vi "Event-Driven State Machine - Inject Error.vi"() -> ()   [LabVIEW 2020]
uses:
  support/States.ctl
  support/State Machine Data.ctl
  <vilib>/DAQmx/read.llb/DAQmx Read (Analog 2D DBL NChan NSamp).vi
  <vilib>/DAQmx/write.llb/DAQmx Write (Analog DBL 1Chan 1Samp).vi
  <vilib>/DAQmx/create/channels.llb/DAQmx Create Channel (AI-Voltage-Basic).vi
  <vilib>/DAQmx/configure/timing.llb/DAQmx Timing (Sample Clock).vi
  <vilib>/DAQmx/miscellaneous.llb/DAQmx Fill In Error Info.vi
  <vilib>/Utility/file.llb/Write Delimited Spreadsheet (DBL).vi
  <vilib>/DAQmx/create/channels.llb/DAQmx Create Channel (AO-Voltage-Basic).vi
panel:
  in  "AO Voltage Channel":tag="PCI-6221/ao1"
  in  "Generate Stimulus":bool
  out "Threshold exceeded?":bool
  in  "Acquire":bool
  in  "Samples per channel":i32=100
  in  "Sample Rate (Hz)":dbl=1000.0
  in  "AI Voltage Channel":tag="PCI-6221/ai0, PCI-6221/ai2:3"
  in  "Threshold (rms)":dbl=1.0
  in  "Clear":bool
  in  "Exit":bool
  out "Graph":dbl[][](graph)
  # "Analysis"
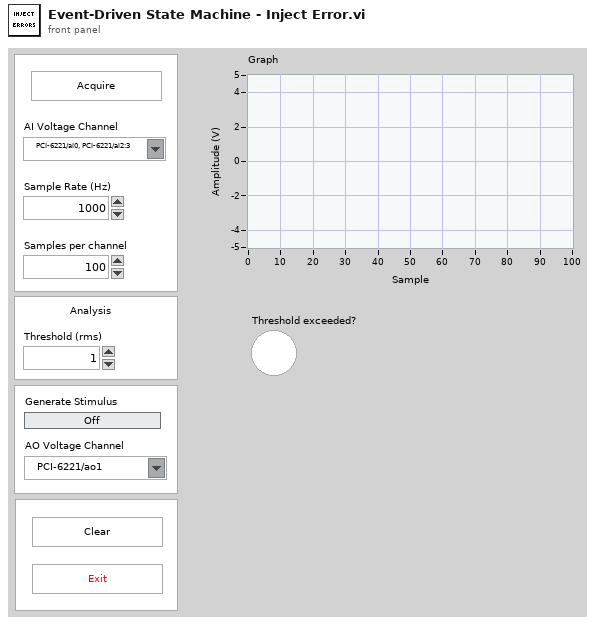
[diagram p1: front panel]
types:
  T1 = typedef "State Machine Data.ctl" = cluster{"Acquisition Data":dbl[][], "Stimulus Value":bool}
  T2 = typedef "States.ctl" = enum16{"Initialize", "Wait for Event", "Acquire", "Analyze", "Log", "Clear", "Update Graph", "Update Stumulus", "Exit"}
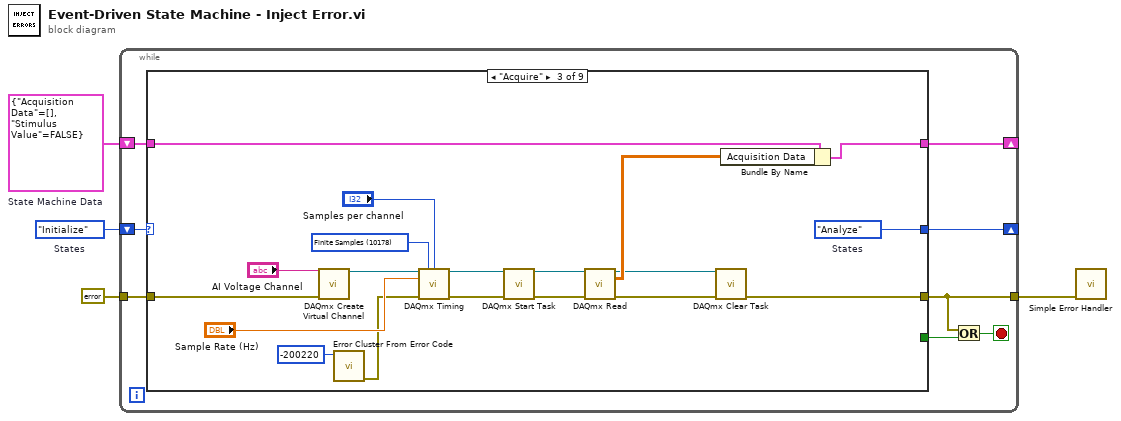
[diagram p0: block diagram]
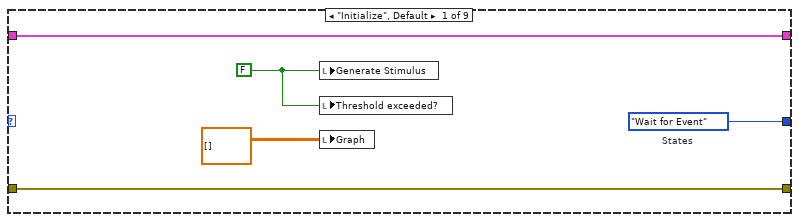
[diagram p2: hidden frame]
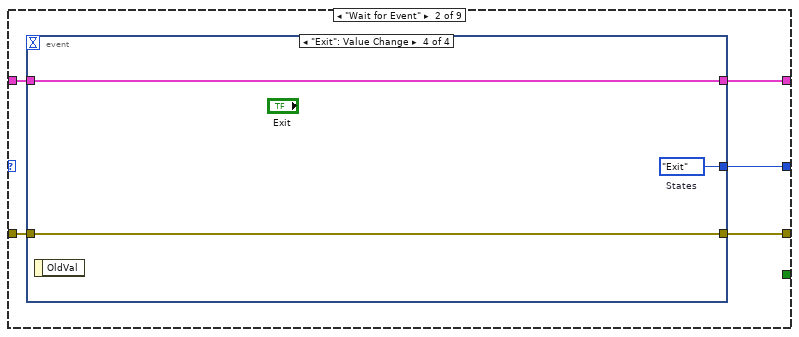
[diagram p3: hidden frame]
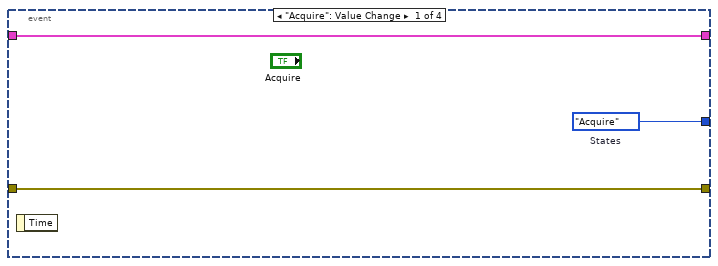
[diagram p4: hidden frame]
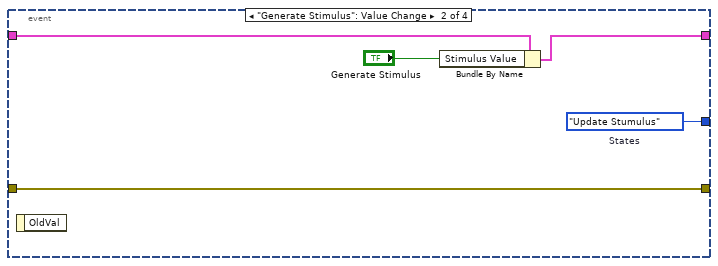
[diagram p5: hidden frame]
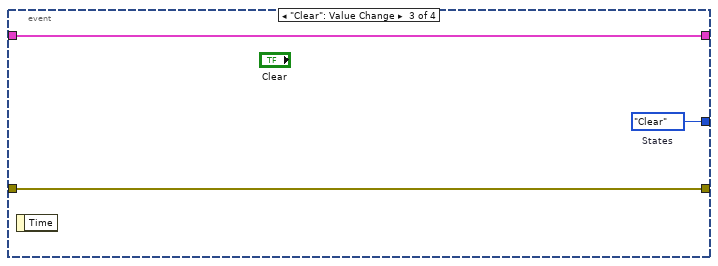
[diagram p6: hidden frame]
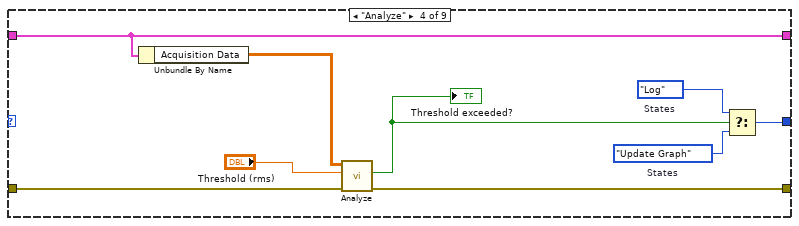
[diagram p7: hidden frame]
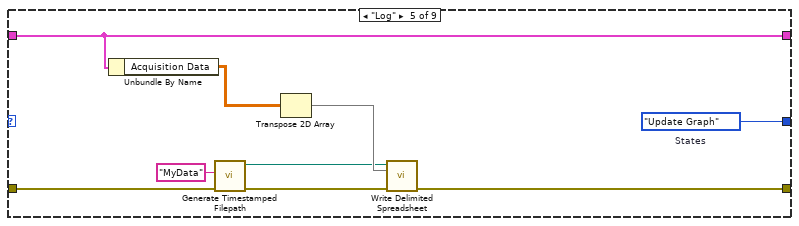
[diagram p8: hidden frame]
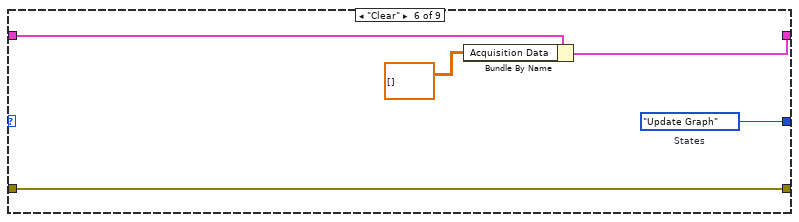
[diagram p9: hidden frame]
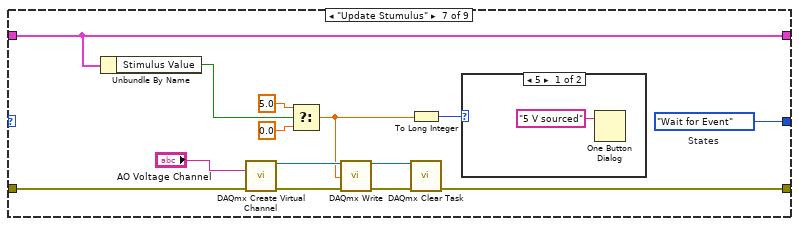
[diagram p10: hidden frame]
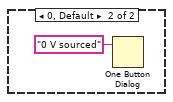
[diagram p11: hidden frame]
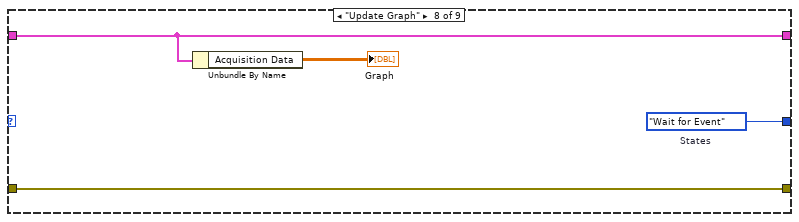
[diagram p12: hidden frame]
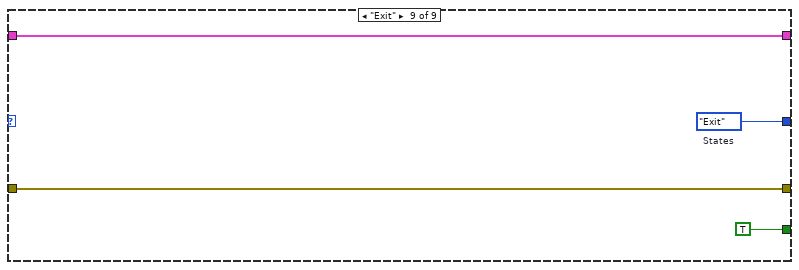
[diagram p13: hidden frame]
diagram:
  w4 = T1 {"Acquisition Data"=[], "Stimulus Value"=FALSE}  # State Machine Data
  w3 = States."Initialize"  # States
  n1 = while {
    tunnel: errorcluster {"status"=FALSE, "code"=0, "source"=""} ("error constant") -> [w11]
    tunnel: [w7] -> w1
    shift-right: [w9] -> _
    shift-left: w4 -> [w10]
    shift-right: [w8] -> _
    shift-left: w3 -> [w12]
    stop <- w6 stop-if-true
    n2 = case shown="\"Acquire\"" w12 {
      tunnel: w11 -> [w17 w20 w55 w63 w72 w78 w80 w97 w101]
      tunnel: [w17 w19 w51 w62 w66 w78 w79 w97 w101] -> w7
      tunnel: [w16 w21 w48 w64 w73 w76 w92 w98 w102] -> w9
      tunnel: w10 -> [w16 w22 w49 w64 w73 w77 w92 w98 w102]
      tunnel: [w15 w18 w50 w58 w65 w74 w81 w96 w99] -> w8
      tunnel: [_ _ _ _ _ _ _ _ TRUE] -> w5
      frame "Initialize", Default {
        w14 = FALSE
        w15 = States."Wait for Event"  # States
        n3 = local write "Generate Stimulus"(w14) -> ()
        n4 = local write "Threshold exceeded?"(w14) -> ()
        n5 = local write "Graph"(dbl[][] []) -> ()
      }
      frame "Wait for Event" {
        n6 = event shown="[3] \"Exit\": Value Change" {
          selector: _ -> [_ _ _ _]
          dyn-events: _ -> [_ _ _ _]
          timeout: _ -> [_ _ _ _]
          tunnel: w22 -> [w25 w30 w33 w35]
          tunnel: [w25 w29 w33 w35] -> w21
          tunnel: w20 -> [w24 w26 w32 w36]
          tunnel: [w24 w26 w32 w36] -> w19
          tunnel: [w23 w27 w31 w34] -> w18
          event "Acquire": Value Change {
            w23 = States."Acquire"  # States
            n7 = event-data() -> ()  [unwired: 1 in, 1 out]
          }
          event "Generate Stimulus": Value Change {
            w27 = States."Update Stumulus"  # States
            n8 = event-data() -> ()  [unwired: 1 in, 1 out]
            n9 = Bundle By Name(cluster=w30, "Stimulus Value"="Generate Stimulus") -> (w29:T1)
          }
          event "Clear": Value Change {
            w31 = States."Clear"  # States
            n10 = event-data() -> ()  [unwired: 1 in, 1 out]
          }
          event "Exit": Value Change {
            w34 = States."Exit"  # States
            n11 = event-data() -> ()  [unwired: 1 in, 1 out]
          }
        }
      }
      frame "Acquire" {
        w47 = 10178 items=["Finite Samples"=10178, "Continuous Samples"=10123, "Hardware Timed Single Point"=12522] ("sample mode")
        w50 = States."Analyze"  # States
        n12 = call-poly <vilib>:"DAQmx Create Virtual Channel.vi"("physical channels"="AI Voltage Channel", "error in"=w55) -> ("task out"=w42:refnum<k21>)  [unwired: 12 in, 1 out]
        n13 = call <vilib>:"Error Cluster From Error Code.vi"("error code (0)"=-200220) -> ("error out"=w37:errorcluster)  [unwired: 8 in]
        n14 = call-poly <vilib>:"DAQmx Timing.vi"("task/channels in"=w42, "sample mode"=w47, "samples per channel"="Samples per channel", "rate"="Sample Rate (Hz)", "error in"=w37) -> ("task out"=w41:refnum<k21>, "error out"=w54:errorcluster)  [unwired: 9 in]
        n15 = call <vilib>:"DAQmx Start Task.vi"("task/channels in"=w41, "error in"=w54) -> ("task out"=w40:refnum<k21>, "error out"=w53:errorcluster)  [unwired: 12 in]
        n16 = call-poly <vilib>:"DAQmx Read.vi"("task/channels in"=w40, "error in"=w53) -> ("task out"=w39:refnum<k21>, "data"=w43:dbl[][], "error out"=w52:errorcluster)  [unwired: 11 in]
        n17 = call <vilib>:"DAQmx Clear Task.vi"("task in"=w39, "error in"=w52) -> ("error out"=w51:errorcluster)  [unwired: 13 in]
        n18 = Bundle By Name(cluster=w49, "Acquisition Data"=w43) -> (w48:T1)
      }
      frame "Analyze" {
        w59 = States."Update Graph"  # States
        w60 = States."Log"  # States
        n19 = Unbundle By Name(w64) -> ("Acquisition Data"=w61:dbl[][])
        n20 = call "Analyze.vi"("Error In"=w63, "Treshold (rms)"="Threshold (rms)", "N-Channel Data (2D DBL)"=w61) -> ("Error Out"=w62:errorcluster, "Threshold exceeded?"=w56:bool)  [unwired: 5 in, 2 out]
        "Threshold exceeded?" <- w56
        n21 = Select(t=w60, s=w56, f=w59) -> (s? t:f=w58:T2)
      }
      frame "Log" {
        w65 = States."Update Graph"  # States
        n22 = Unbundle By Name(w73) -> ("Acquisition Data"=w70:dbl[][])
        n23 = call "Generate Timestamped Filepath.vi"("Error In"=w72, "appended filename"="MyData") -> ("Error Out"=w67:errorcluster, "timestamped relative filepath"=w68:path)  [unwired: 8 in]
        n24 = Transpose 2D Array(2D array=w70) -> (transposed array=w69:dbl[][])
        n25 = call-poly <vilib>:"Write Delimited Spreadsheet.vi"("file path (dialog if empty)"=w68, "2D data"=w69, "error in (no error)"=w67) -> ("error out"=w66:errorcluster)  [unwired: 11 in, 1 out]
      }
      frame "Clear" {
        w74 = States."Update Graph"  # States
        n26 = Bundle By Name(cluster=w77, "Acquisition Data"=dbl[][] []) -> (w76:T1)
      }
      frame "Update Stumulus" {
        w81 = States."Wait for Event"  # States
        n27 = Unbundle By Name(w92) -> ("Stimulus Value"=w82:bool)
        n28 = call-poly <vilib>:"DAQmx Create Virtual Channel.vi"("physical channels"="AO Voltage Channel", "error in"=w80) -> ("task out"=w89:refnum<k21>, "error out"=w88:errorcluster)  [unwired: 12 in]
        n29 = Select(t=5.0, s=w82, f=0.0) -> (s? t:f=w84:dbl)
        n30 = call-poly <vilib>:"DAQmx Write.vi"("task/channels in"=w89, "data"=w84, "error in"=w88) -> ("task out"=w87:refnum<k21>, "error out"=w86:errorcluster)  [unwired: 10 in, 1 out]
        n31 = To Long Integer(number=w84) -> (32bit integer=w83:i32)
        n32 = call <vilib>:"DAQmx Clear Task.vi"("task in"=w87, "error in"=w86) -> ("error out"=w79:errorcluster)  [unwired: 13 in]
        n33 = case shown="5" w83 {
          frame 5 {
            n34 = One Button Dialog(message="5 V sourced") -> ()  [unwired: 1 in, 1 out]
          }
          frame 0, Default {
            n35 = One Button Dialog(message="0 V sourced") -> ()  [unwired: 1 in, 1 out]
          }
        }
      }
      frame "Update Graph" {
        w96 = States."Wait for Event"  # States
        n36 = Unbundle By Name(w98) -> ("Acquisition Data"=→"Graph":dbl[][])
      }
      frame "Exit" {
        w99 = States."Exit"  # States
      }
    }
    n37 = Or(x=w7, y=w5) -> (x .or. y?=w6:bool)
  }
  n38 = call <vilib>:"Simple Error Handler.vi"("error in (no error)"=w1) -> ()  [unwired: 4 in, 5 out]
